vi "GetFieldFromProtobufIndexGreeter_MessageA_oneof_a.vi"(1 "protobuf index":i32) -> (0 "oneof field name":string)   [LabVIEW 2019, in "Generated_server.lvlib" / "Greeter_MessageA_oneof_a.lvclass"]
uses:
  Greeter_MessageA_oneof_a.lvclass
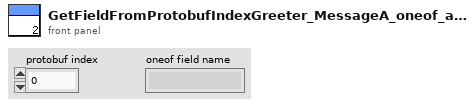
[diagram p1: front panel]
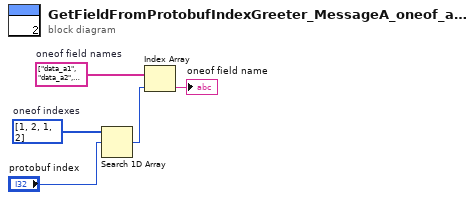
[diagram p0: block diagram]
diagram:
  w5 = string[] ["data_a1", "data_a2", "data_a1", "data_a2"]  # oneof field names
  w4 = i32[] [1, 2, 1, 2]  # oneof indexes
  n1 = Search 1D Array(1D array=w4, element="protobuf index") -> (index of element=w2:i32)  [unwired: 1 in]
  n2 = Index Array(array=w5, index=w2) -> (element=→"oneof field name":string)
